vi "Inverse Transmission Model v3.vi"(7 "Sensors":T1, 10 "Torque Reference":dbl) -> (1 "Motor Command":dbl, 3 "R_tau":dbl)   [LabVIEW 2018]
uses:
  Sensor Data.ctl
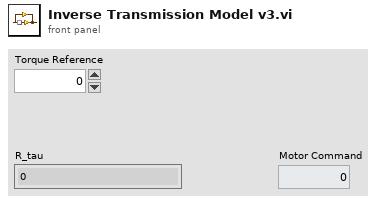
[diagram p1: front panel]
types:
  T1 = typedef "Sensor Data.ctl" = cluster{"Motor Current":dbl, "Motor Velocity":dbl, "Ankle Encoder Angle":dbl, "GRF L":dbl, "GRF R":dbl, "Index pulse?":bool, "Roll":dbl, "Pitch":dbl, "Yaw":dbl, "Thigh Angle":dbl}
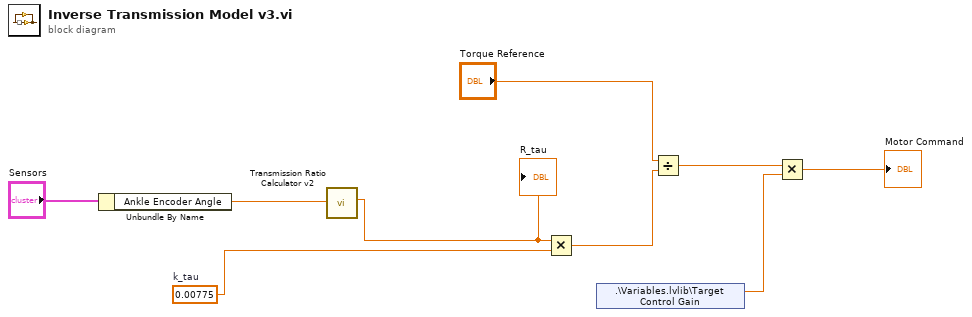
[diagram p0: block diagram]
diagram:
  w7 = 0.00775  # k_tau
  n1 = Unbundle By Name("Sensors") -> ("Ankle Encoder Angle"=w5:dbl)
  n2 = call "Transmission Ratio Calculator v2.vi"("Ankle Angle"=w5) -> ("R_tau"=w8:dbl)  [unwired: 10 in]
  "R_tau" <- w8
  n3 = Multiply(x=w8, y=w7) -> (x*y=w6:dbl)
  n4 = shared-variable ".\\Variables.lvlib\\Target Control Gain"() -> (w2:dbl)  [unwired: 1 in, 1 out]
  n5 = Divide(x="Torque Reference", y=w6) -> (x/y=w4:dbl)
  n6 = Multiply(x=w4, y=w2) -> (x*y=→"Motor Command":dbl)
